vi "EnFlo_Tun_Heater_Control.vi"(1 "Ch Names":string[](array[string]), 2 "Heaters Just Enabled":bool, 3 "Values":dbl[](array[numeric]) format="%.2f") -> ()   [LabVIEW 2012]
uses:
  ADAM Client/Sub VIs/ADAM Controls/Search_mode.ctl
  ADAM_Global.vi
  <vilib>/Analysis/baseanly.llb/Mean (DBL).vi
  <vilib>/Analysis/NI_AALPro.lvlib
  <vilib>/Analysis/NI_AALBase.lvlib
panel:
  out "Read Values OK":bool
  out "History Out":dbl[](array[numeric])
  out "Current Temp":dbl
  out "Setpoint":dbl
  out "Large Error?":bool
  out "Error Range":dbl
  in  "Index To Display":i32
  in  "Derivative History Change":i32=60
  out "Feedback Temperature":string
  in  "Use Change Coeff if error above:":dbl=5.0 format="%_3g"
  in  "Minimum Power Change in %":dbl=0.08
  in  "Total History":i32=200
  out "Proportional Term":dbl format="%#.1f"
  out "Control Sum":dbl format="%#.1f"
  out "Differential Term":dbl format="%#.1f"
  in  "Derivative History":i32=60
  out "Integral Term":dbl format="%#.1f"
  # "This is the Max - Min error for the Total History"
  # "When Changing\nSetpoint"
  # "When running at\nSteady Cond"
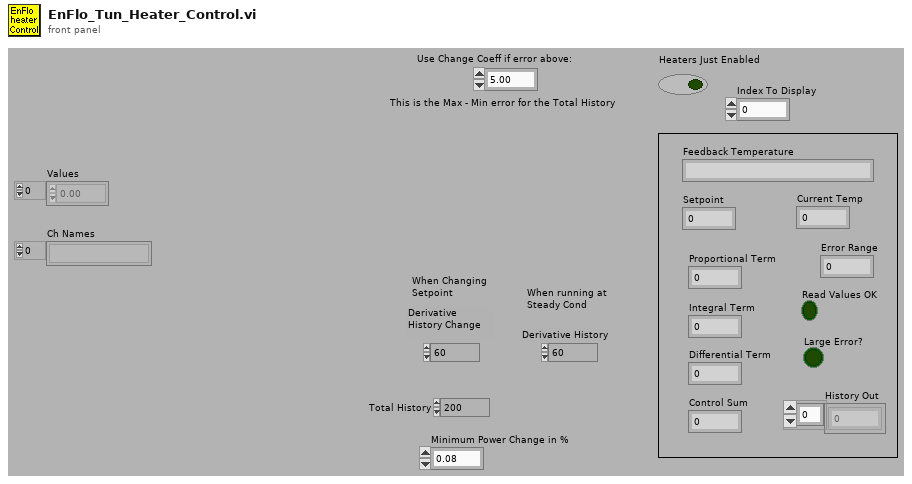
[diagram p1: front panel]
types:
  T1 = enum16{"On", "Off", "Always On", "Always Off", "Delete"}
  T2 = typedef "Search_mode.ctl" = enum16{"Between times", "All Times"}
  T3 = typedef "Ch_description_ADAM.ctl" = cluster{"Ch Name":string, "Type":T4, "Function":T5, "Ch State":T6, "Calibration type":T7, "A":dbl, "B":dbl, "C":dbl, "D":dbl, "Comments":string, "Address":T8, "String":string, "Duty":u16}
  T4 = typedef "Module_type_ADAM.ctl" = string
  T5 = typedef "Function_ADAM.ctl" = enum16{"Analogue Input", "Digital Input", "Event counter", "Event rate", "Analogue Output", "Digital Output", "Relay Output"}
  T6 = typedef "Channel_State.ctl" = enum16{"On", "Off", "Always On", "Always Off"}
  T7 = typedef "Calib_type_ADAM.ctl" = enum16{"Raw", "Bx + A", "Cx^2 + Bx + A", "Dx^3 + Cx^2 + Bx + A", "In Band", "Hi-Tec Q", "Hi-Tec M_dot", "Text"}
  T8 = typedef "Address.ctl" = cluster{"Main":i32, "Ch.":i32, "Sub":i32, "Port Name":string}
  T9 = cluster{"Centre Times":dbl[], "Output array":dbl[]}
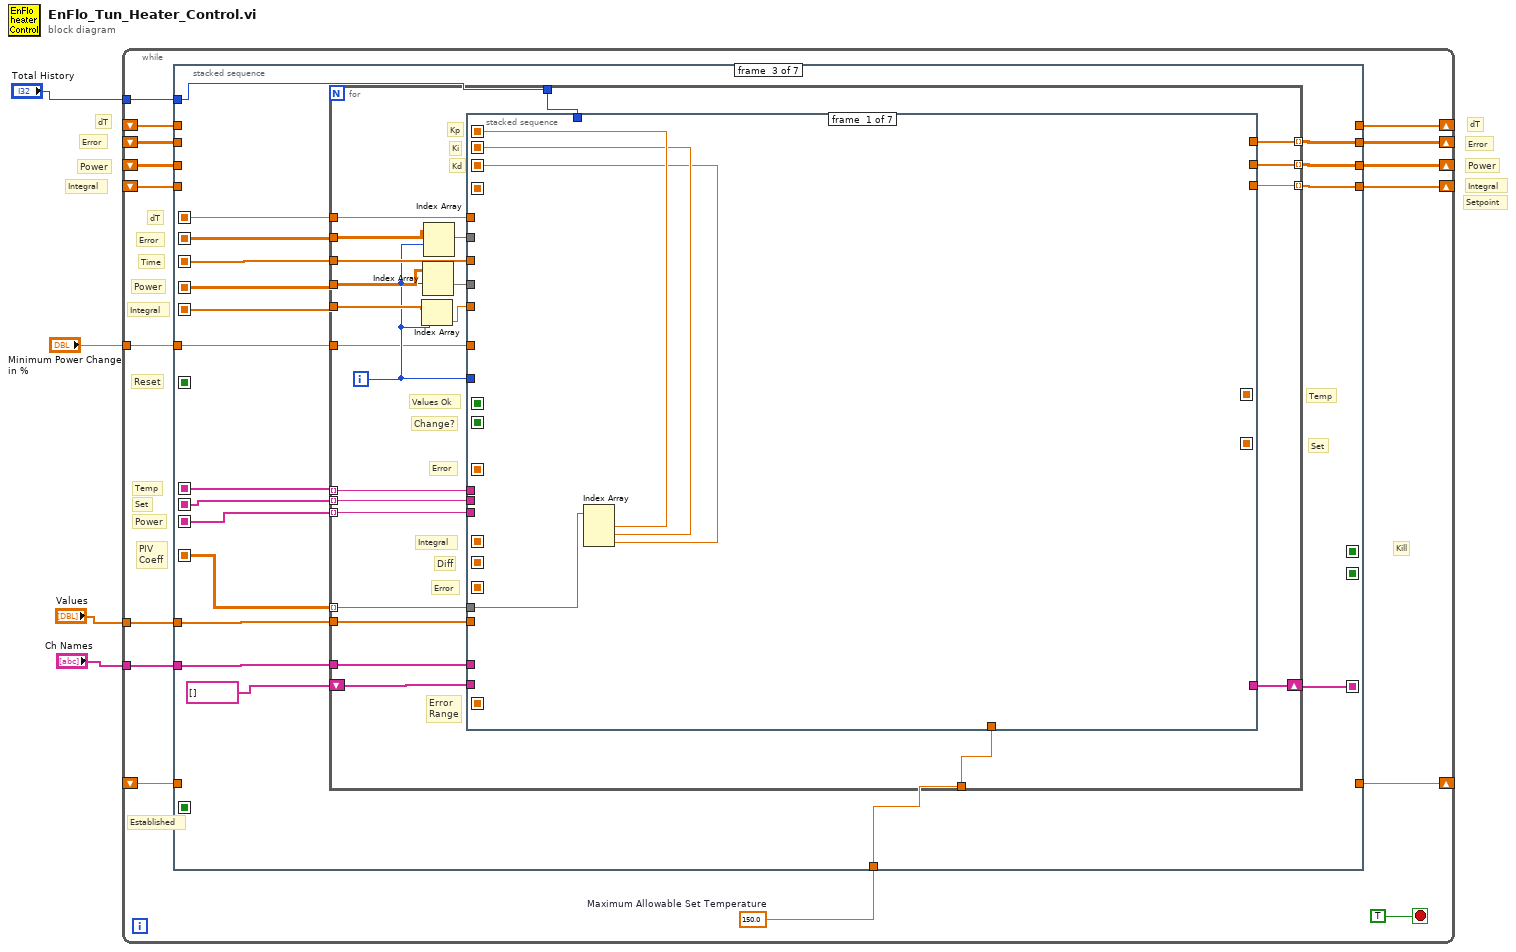
[diagram p0: block diagram]
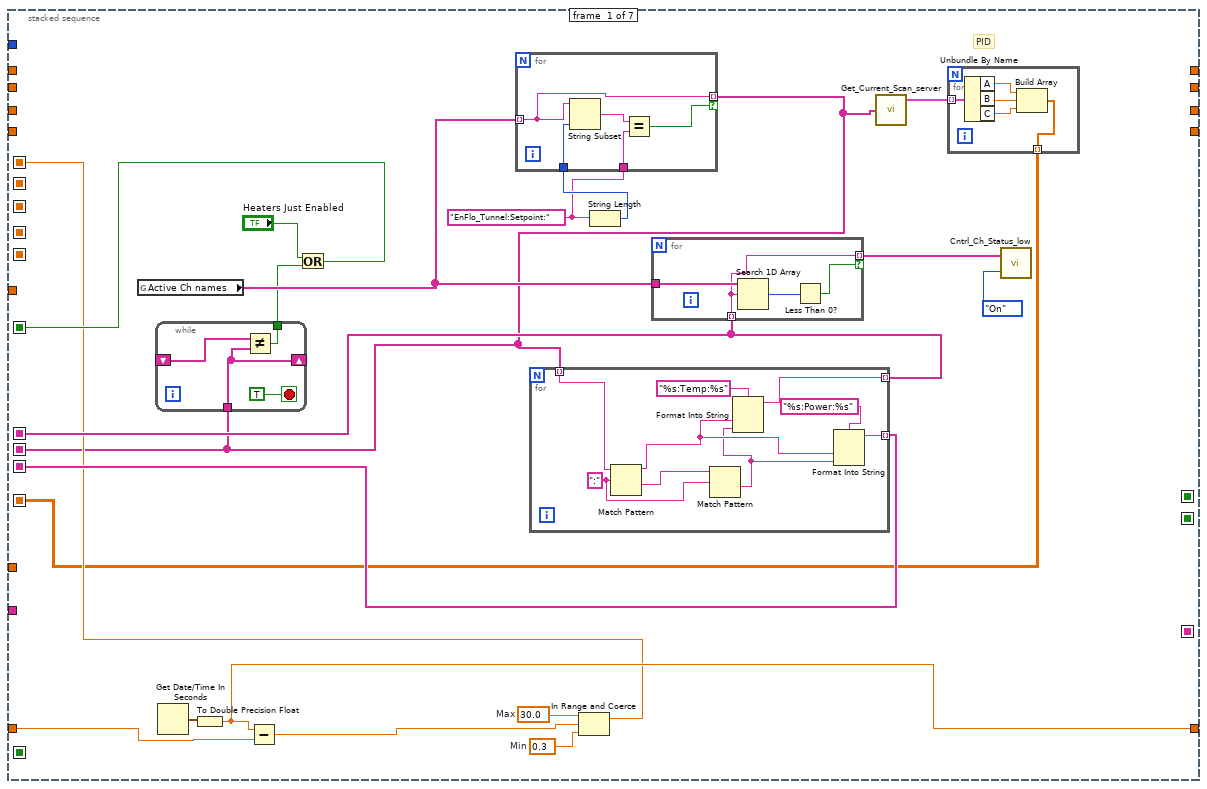
[diagram p2: hidden frame]
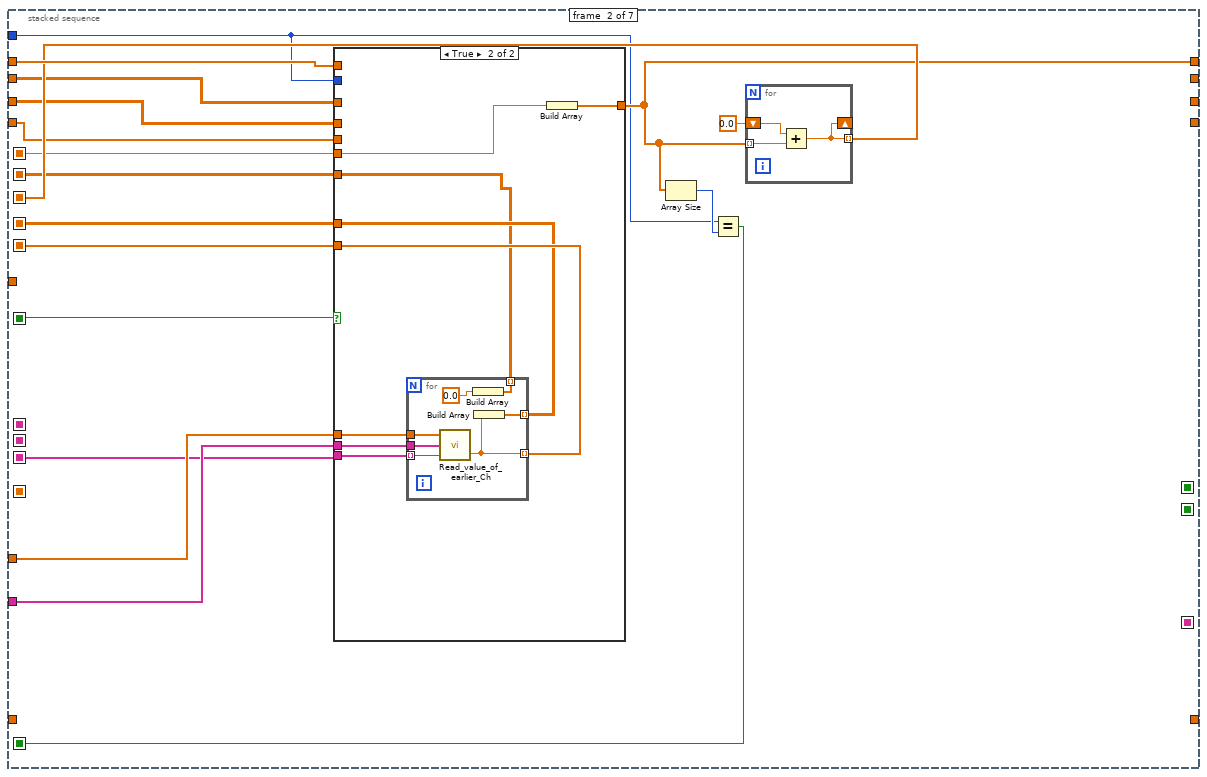
[diagram p3: hidden frame]
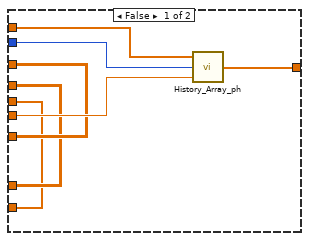
[diagram p4: hidden frame]
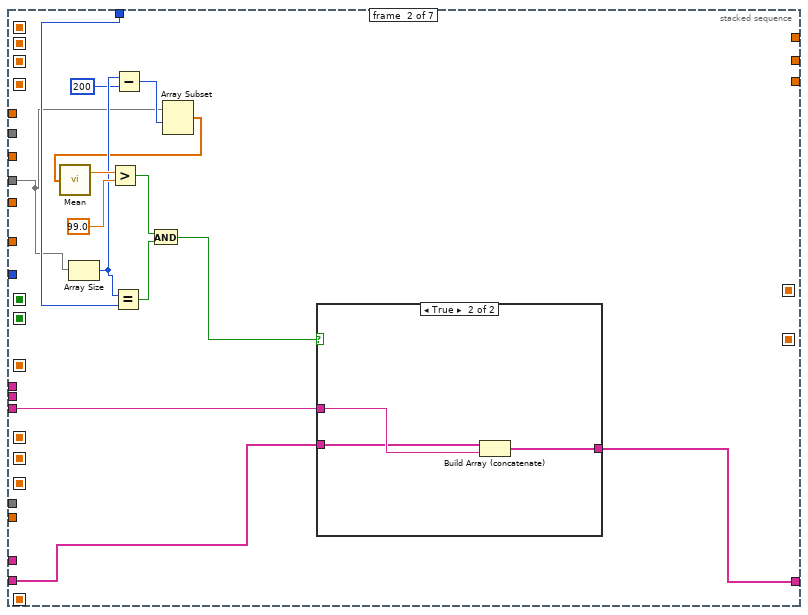
[diagram p5: hidden frame]
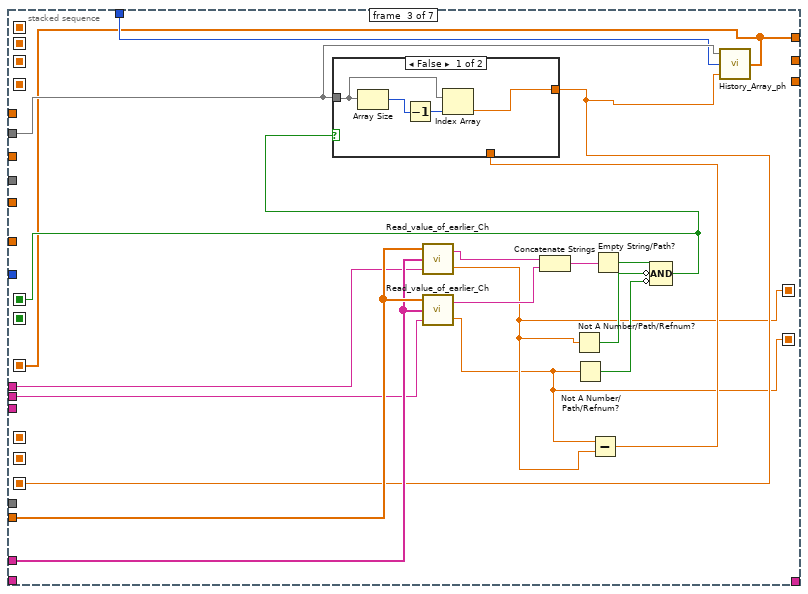
[diagram p7: hidden frame]
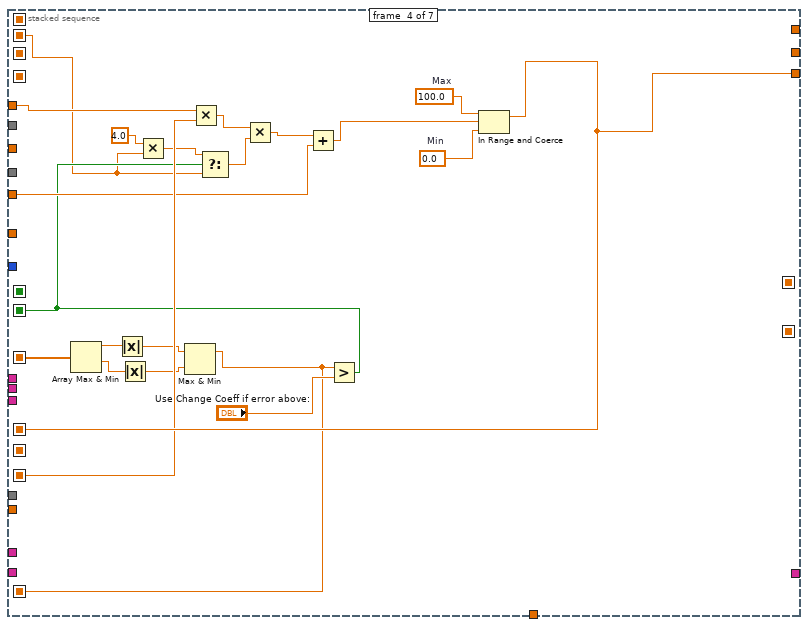
[diagram p9: hidden frame]
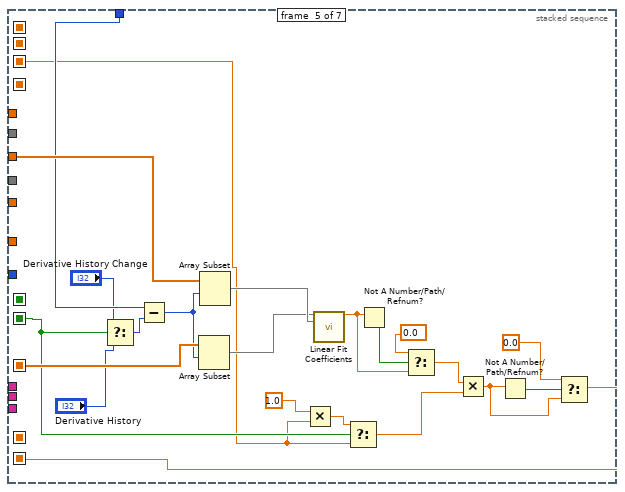
[diagram p10: hidden frame]
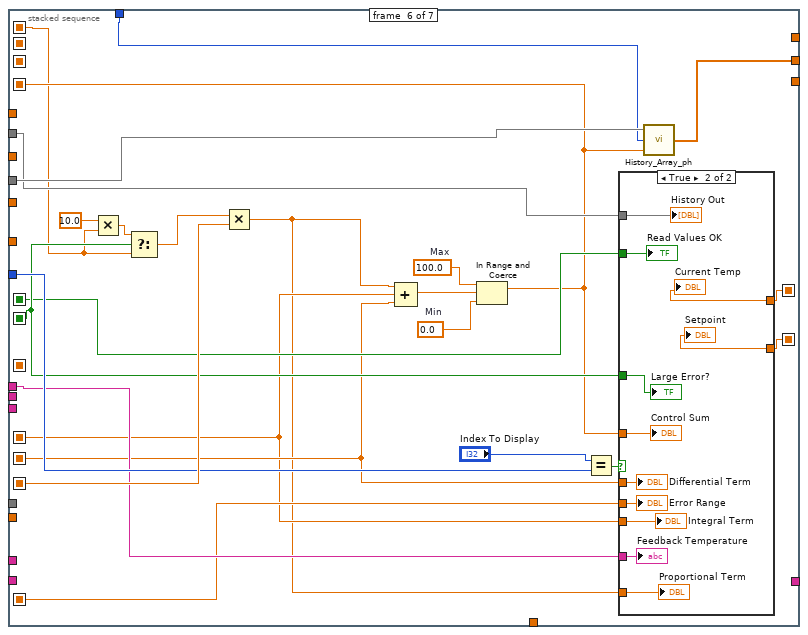
[diagram p11: hidden frame]
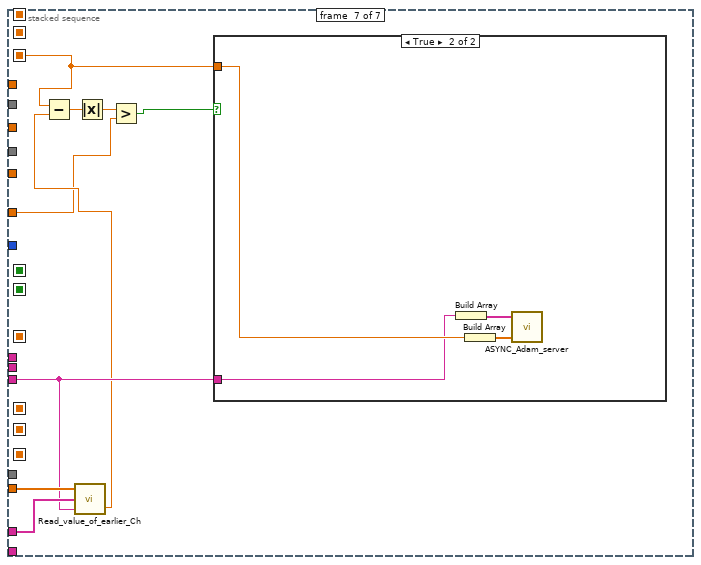
[diagram p13: hidden frame]
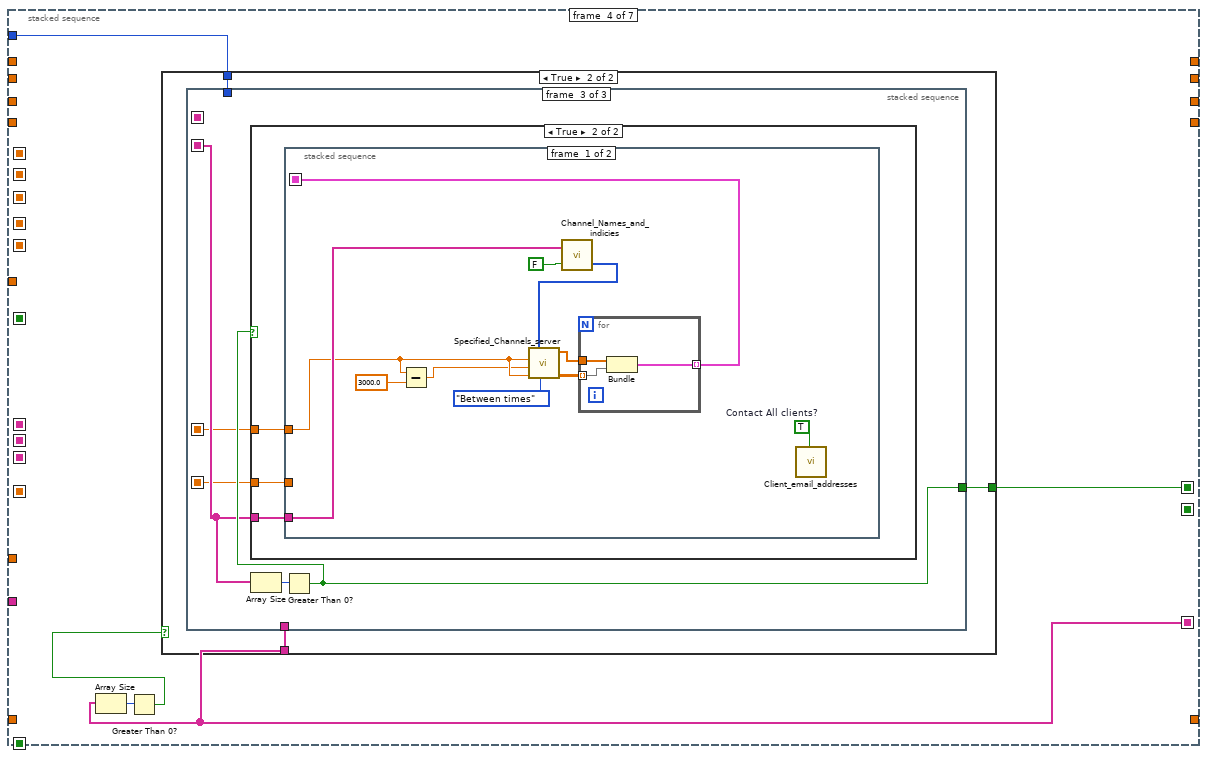
[diagram p15: hidden frame]
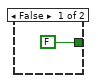
[diagram p16: hidden frame]
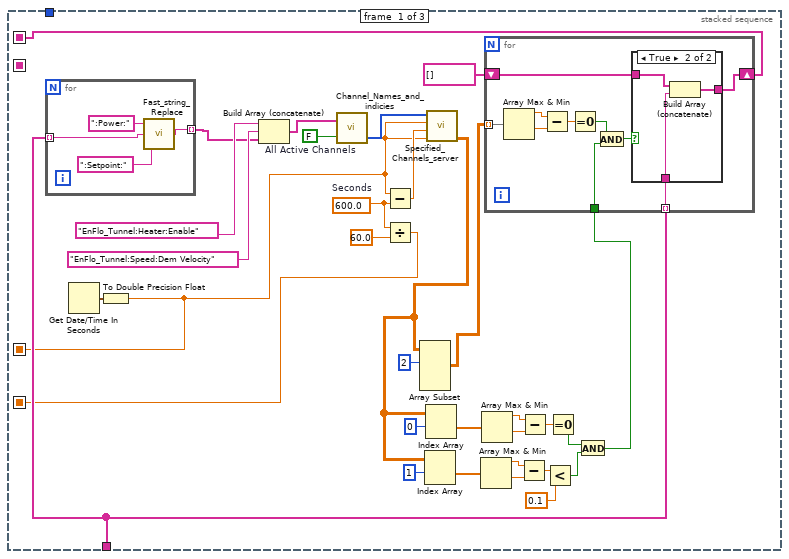
[diagram p17: hidden frame]
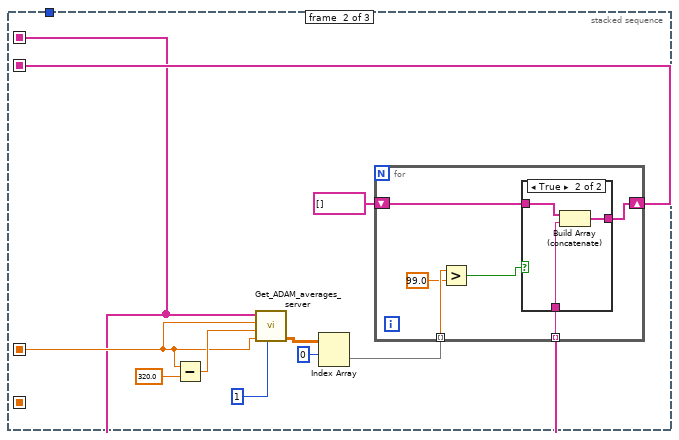
[diagram p19: hidden frame]
diagram:
  # "Integral"
  # "Power"
  # "Error"
  # "dT"
  # "Setpoint"
  # "Power"
  # "Integral"
  # "Error"
  # "dT"
  n1 = while {
    shift-right: [w18] -> _
    shift-left: _ -> [w19]
    shift-right: [w14] -> _
    shift-left: _ -> [w17]
    shift-right: [w16] -> _
    shift-left: _ -> [w15]
    shift-right: [w12] -> _
    shift-left: _ -> [w13]
    shift-right: [w10] -> _
    shift-left: _ -> [w11]
    tunnel: "Total History" -> [w9]
    tunnel: "Ch Names" -> [w7]
    tunnel: "Values" -> [w6]
    tunnel: "Minimum Power Change in %" -> [w5]
    stop <- TRUE stop-if-true
    w8 = 150.0  # Maximum Allowable Set Temperature
    # "Established"
    # "PIV\nCoeff"
    # "dT"
    # "Integral"
    # "Power"
    # "Error"
    # "Reset"
    # "Kill"
    # "Power"
    # "Set"
    # "Temp"
    # "Time"
    n2 = stacked-sequence {
      seq-local: [_ w82 _ _ _ _ _] -> [_ _ w128 _ _ _ _]
      seq-local: [w31 _ _ _ _ _ _] -> [_ _ w125 _ _ w452 _]
      seq-local: [w22 _ _ _ _ _ _] -> [_ _ w124 _ _ w451 _]
      seq-local: [w38 _ _ _ _ _ _] -> [_ w72 w123 _ _ w454 _]
      seq-local: [_ _ w120 _ _ _ _] -> [_ _ _ w292 _ _ _]
      seq-local: [_ _ _ w290 _ _ _] -> [_ _ _ _ w413 _ _]
      seq-local: [_ _ _ _ w414 _ _] -> [_ _ _ _ _ _ w495]
      seq-local: [w25 _ _ _ _ _ _] -> [_ w81 w116 _ _ _ _]
      seq-local: [w26 _ _ _ _ _ _] -> [_ w84 _ _ _ _ _]
      seq-local: [_ w80 _ _ _ _ _] -> [_ _ w113 _ _ _ _]
      seq-local: [_ w78 _ _ _ _ _] -> [_ _ w114 _ _ _ _]
      seq-local: [_ w76 _ _ _ _ _] -> [_ _ w115 _ _ _ _]
      seq-local: [w23 _ _ _ _ _ _] -> [_ _ w111 _ _ _ _]
      seq-local: [_ w68 _ _ _ _ _] -> [_ _ _ _ _ w443 _]
      tunnel: w19 -> [_ w85 _ _ _ _ _]
      tunnel: [_ w71 _ _ _ _ _] -> w18
      tunnel: w17 -> [_ w79 _ _ _ _ _]
      tunnel: [w32 _ _ _ _ _ _] -> w16
      tunnel: w15 -> [w34 _ _ _ _ _ _]
      tunnel: [_ _ w129 _ _ _ _] -> w14
      tunnel: w13 -> [_ w77 _ _ _ w453 _]
      tunnel: [_ _ w127 _ _ _ _] -> w12
      tunnel: w11 -> [_ w75 _ _ _ _ _]
      tunnel: [_ _ w126 _ _ _ _] -> w10
      tunnel: w9 -> [_ w69 w117 w293 w415 _ _]
      tunnel: w8 -> [_ _ w121 _ w407 _ _]
      tunnel: w7 -> [_ w73 w119 _ w410 w449 _]
      tunnel: w6 -> [_ w74 w118 _ w409 w450 _]
      tunnel: w5 -> [_ _ w112 _ _ w446 _]
      frame #0 {
        w36 = 0.3  # Min
        w35 = 30.0  # Max
        w39 = "EnFlo_Tunnel:Setpoint:"
        # "PID"
        n3 = global read "ADAM_Global.vi" "Active Ch names"() -> (w29:string[])
        n4 = Get Date/Time In Seconds() -> (seconds since 1Jan1904=w37:timestamp)
        n5 = To Double Precision Float(number=w37) -> (double precision float=w32:dbl)
        n6 = Subtract(x=w32, y=w34) -> (x-y=w33:dbl)
        n7 = In Range and Coerce(upper limit=w35, x=w33, lower limit=w36) -> (coerced(x)=w25:dbl)  [unwired: 1 out]
        n8 = String Length(string=w39) -> (length=w40:i32)
        n9 = for {
          tunnel: w29 -> [w55] mode=indexing
          tunnel: w40 -> [w58]
          tunnel: w39 -> [w57]
          tunnel: [w55] -> w22 mode=indexing if=w54
          n10 = String Subset(string=w55, length (rest)=w58) -> (substring=w56:string)  [unwired: 1 out]
          n11 = Equal?(x=w56, y=w57) -> (x = y?=w54:bool)
        }
        n12 = while {
          shift-right: [w49] -> _
          shift-left: _ -> [w48]
          tunnel: w22 -> [w49]
          tunnel: [w47] -> w27
          stop <- TRUE stop-if-true
          n13 = Not Equal?(x=w48, y=w49) -> (x != y?=w47:bool)
        }
        n14 = Or(x="Heaters Just Enabled", y=w27) -> (x .or. y?=w26:bool)
        n15 = for {
          tunnel: w22 -> [w59] mode=indexing
          tunnel: [w60] -> w38 mode=indexing
          tunnel: [w61] -> w31 mode=indexing
          w66 = ":" ("regular expression")
          n16 = Match Pattern(string=w59, regular expression=w66) -> (before substring=w63:string, after substring=w67:string)  [unwired: 3 out]
          n17 = Match Pattern(string=w67, regular expression=w66) -> (after substring=w62:string)  [unwired: 4 out]
          n18 = Format Into String(format string="%s:Temp:%s", w63, w62) -> (resulting string=w61:string)  [unwired: 2 in, 1 out]
          n19 = Format Into String(format string="%s:Power:%s", w63, w62) -> (resulting string=w60:string)  [unwired: 2 in, 1 out]
        }
        n20 = for {
          tunnel: w31 -> [w52] mode=indexing
          tunnel: w29 -> [w53]
          tunnel: [w52] -> w21 mode=indexing if=w50
          n21 = Search 1D Array(1D array=w53, element=w52) -> (index of element=w51:i32)  [unwired: 1 in]
          n22 = Less Than 0?(x=w51) -> (x < 0?=w50:bool)
        }
        n23 = call "Get_Current_Scan_server.vi"("Desired Channels"=w22) -> ("Ch Description Array"=w24:T3[])  [unwired: 2 out]
        n24 = for {
          tunnel: w24 -> [w45] mode=indexing
          tunnel: [w41] -> w23 mode=indexing
          n25 = Unbundle By Name(w45) -> ("A"=w44:dbl, "B"=w43:dbl, "C"=w42:dbl)
          n26 = Build Array(w44, w43, w42) -> (w41:dbl[])
        }
        n27 = call "Cntrl_Ch_Status_low.vi"("Mode"=T1."On", "Channel names"=w21) -> ()  [unwired: 1 out]
      }
      frame #1 {
        n28 = case shown="True" w84 {
          tunnel: [w95 w103] -> w71
          tunnel: w85 -> [w94 _]
          tunnel: w69 -> [w93 _]
          tunnel: w81 -> [w92 w102]
          tunnel: [w91 w96] -> w80
          tunnel: w79 -> [w91 _]
          tunnel: [w90 w97] -> w78
          tunnel: w77 -> [w90 _]
          tunnel: [w89 w98] -> w76
          tunnel: w75 -> [w89 _]
          tunnel: w74 -> [_ w101]
          tunnel: w73 -> [_ w100]
          tunnel: w72 -> [_ w99]
          frame False {
            n29 = call "History_Array_ph.vi"("Current Value"=w92, "Desired Length"=w93, "History In"=w94) -> ("History Out"=w95:dbl[])
          }
          frame True {
            n30 = for {
              tunnel: w101 -> [w110]
              tunnel: w100 -> [w109]
              tunnel: w99 -> [w108] mode=indexing
              tunnel: [w104] -> w98 mode=indexing
              tunnel: [w107] -> w97 mode=indexing
              tunnel: [w105] -> w96 mode=indexing
              n31 = call "Read_value_of_earlier_Ch.vi"("Desired Ch to Read"=w108, "Ch names"=w109, "Present scan array"=w110) -> ("Value"=w104:dbl)  [unwired: 1 in, 1 out]
              n32 = Build Array(0.0) -> (w105:dbl[])
              n33 = Build Array(w104) -> (w107:dbl[])
            }
            n34 = Build Array(w102) -> (w103:dbl[])
          }
        }
        n35 = Array Size(array=w71) -> (size(s)=w70:i32)
        n36 = Equal?(x=w69, y=w70) -> (x = y?=w68:bool)
        n37 = for {
          shift-right: [w87] -> _
          shift-left: 0.0 ("element") -> [w88]
          tunnel: [w87] -> w82 mode=indexing
          tunnel: w71 -> [w86] mode=indexing
          n38 = Add(x=w88, y=w86) -> (x+y=w87:dbl)
        }
      }
      frame #2 {
        # "Temp"
        # "Set"
        n39 = for {
          tunnel: w118 -> [w137]
          tunnel: w119 -> [w136]
          tunnel: [w152] -> w129 mode=indexing
          tunnel: w113 -> [w140]
          tunnel: w116 -> [w151]
          tunnel: w128 -> [w142]
          tunnel: [w150] -> w127 mode=indexing
          tunnel: w114 -> [w141]
          tunnel: [w149] -> w126 mode=indexing
          tunnel: w115 -> [w143]
          tunnel: w125 -> [w148] mode=indexing
          tunnel: w124 -> [w135] mode=indexing
          tunnel: w123 -> [w147] mode=indexing
          shift-right: [w145] -> w120
          shift-left: string[] [] -> [w146]
          tunnel: w121 -> [w144]
          tunnel: w117 -> [w139]
          tunnel: w112 -> [w131]
          tunnel: w111 -> [w130] mode=indexing
          i -> [w138]
          # "Kd"
          # "Ki"
          # "Kp"
          # "Values Ok"
          # "Error\nRange"
          # "Change?"
          # "Integral"
          # "Error"
          # "Error"
          # "Diff"
          n40 = Index Array(array=w143, index=w138) -> (element=w134:dbl)
          n41 = Index Array(array=w141, index (row)=w138) -> (element=w132:dbl[])  [unwired: 1 in]
          n42 = Index Array(array=w140, index (row)=w138) -> (element=w133:dbl[])  [unwired: 1 in]
          n43 = stacked-sequence {
            seq-local: [_ _ _ _ w235 _ _] -> [_ _ _ _ _ w246 _]
            seq-local: [_ _ w178 _ _ _ _] -> [_ _ _ w217 _ w265 _]
            seq-local: [_ _ w177 _ _ _ _] -> [_ _ _ w215 w230 _ _]
            seq-local: [_ _ _ w218 _ _ _] -> [_ _ _ _ _ w245 _]
            seq-local: [_ _ _ _ _ w247 _] -> [_ _ _ _ _ _ w282]
            seq-local: [_ _ w179 _ _ _ _] -> [_ _ _ _ _ w248 _]
            seq-local: [_ _ _ w213 _ _ _] -> [_ _ _ _ w225 w252 _]
            seq-local: [_ _ _ w202 _ _ _] -> [_ _ _ _ _ w253 _]
            seq-local: [_ _ w176 _ _ _ _] -> [_ _ _ _ _ w250 _]
            seq-local: [_ _ w175 _ _ _ _] -> [_ _ _ _ _ w251 _]
            seq-local: [w155 _ _ _ _ _ _] -> [_ _ _ _ _ w243 _]
            seq-local: [w154 _ _ _ _ _ _] -> [_ _ _ w200 _ _ _]
            seq-local: [w153 _ _ _ _ _ _] -> [_ _ _ _ w221 _ _]
            tunnel: w137 -> [_ _ w192 _ _ _ w285]
            tunnel: w136 -> [_ _ w191 _ _ _ w284]
            tunnel: [_ _ w177 _ _ _ _] -> w152
            tunnel: w133 -> [_ _ w181 _ _ w249 _]
            tunnel: w151 -> [_ _ _ w201 _ _ _]
            tunnel: w142 -> [_ _ _ _ w232 _ _]
            tunnel: [_ _ _ _ _ w261 _] -> w150
            tunnel: w132 -> [_ w158 _ _ _ w260 _]
            tunnel: [_ _ _ w218 _ _ _] -> w149
            tunnel: w134 -> [_ _ _ w216 _ _ _]
            tunnel: w148 -> [_ _ w182 _ _ w254 _]
            tunnel: w135 -> [_ _ w183 _ _ _ _]
            tunnel: w147 -> [_ w165 _ _ _ _ w283]
            tunnel: w146 -> [_ w164 _ _ _ _ _]
            tunnel: [_ w163 _ _ _ _ _] -> w145
            tunnel: w144 -> [_ _ _ _ _ _ _]
            tunnel: w139 -> [_ w162 w180 _ w227 w259 _]
            tunnel: w138 -> [_ _ _ _ _ w256 _]
            tunnel: w131 -> [_ _ _ _ _ _ w277]
            tunnel: w130 -> [w156 _ _ _ _ _ _]
            frame #0 {
              n44 = Index Array(array=w156) -> (element #1=w155:dbl, element #2=w154:dbl, element #3=w153:dbl)  [unwired: 3 in]
            }
            frame #1 {
              n45 = Array Size(array=w158) -> (size(s)=w161:i32)
              n46 = Equal?(x=w161, y=w162) -> (x = y?=w168:bool)
              n47 = Subtract(x=w161, y=200) -> (x-y=w159:i32)
              n48 = Array Subset(array=w158, index=w159) -> (w157:dbl[])  [unwired: 1 in]
              n49 = call-poly <vilib>:"Mean.vi"("X"=w157) -> ("mean"=w170:dbl)  [unwired: 1 out]
              n50 = Greater?(x=w170, y=99.0) -> (0:w167:bool)
              n51 = And(x=w167, y=w168) -> (x .and. y?=w166:bool)
              n52 = case shown="True" w166 {
                tunnel: w165 -> [_ w174]
                tunnel: w164 -> [w171 w173]
                tunnel: [w171 w172] -> w163
                frame False {
                }
                frame True {
                  n53 = Build Array (concatenate)(w173, w174) -> (w172:string[])
                }
              }
            }
            frame #2 {
              n54 = call "Read_value_of_earlier_Ch.vi"("Desired Ch to Read"=w182, "Ch names"=w191, "Present scan array"=w192) -> ("Value"=w176:dbl, "Scan comment"=w190:string)  [unwired: 1 in]
              n55 = call "Read_value_of_earlier_Ch.vi"("Desired Ch to Read"=w183, "Ch names"=w191, "Present scan array"=w192) -> ("Value"=w175:dbl, "Scan comment"=w189:string)  [unwired: 1 in]
              n56 = Concatenate Strings(w190, w189) -> (w188:string)
              n57 = Not A Number/Path/Refnum?(number/path/refnum=w176) -> (NaN/Path/Refnum?=w186:bool)
              n58 = Not A Number/Path/Refnum?(number/path/refnum=w175) -> (NaN/Path/Refnum?=w185:bool)
              n59 = Subtract(x=w175, y=w176) -> (x-y=w184:dbl)
              n60 = Empty String/Path?(string/path=w188) -> (empty?=w187:bool)
              n61 = Compound Arithmetic op=AND(w187, invert w186, invert w185) -> (w179:bool)
              n62 = case shown="False" w179 {
                tunnel: w181 -> [w193 _]
                tunnel: [w196 w197] -> w178
                tunnel: w184 -> [_ w197]
                frame False {
                  n63 = Array Size(array=w193) -> (size(s)=w194:i32)
                  n64 = Decrement(x=w194) -> (x-1=w195:i32)
                  n65 = Index Array(array=w193, index=w195) -> (element=w196:dbl)
                }
                frame True {
                }
              }
              n66 = call "History_Array_ph.vi"("Current Value"=w178, "Desired Length"=w180, "History In"=w181) -> ("History Out"=w177:dbl[])
            }
            frame #3 {
              w212 = 0.0  # Min
              w211 = 100.0  # Max
              n67 = Array Max & Min(array=w215) -> (max value=w206:dbl, min value=w205:dbl)  [unwired: 2 out]
              n68 = Absolute Value(x=w206) -> (abs(x)=w203:dbl)
              n69 = Absolute Value(x=w205) -> (abs(x)=w204:dbl)
              n70 = Multiply(x=4.0, y=w200) -> (x*y=w198:dbl)
              n71 = Max & Min(x=w203, y=w204) -> (max(x,y)=w202:dbl)  [unwired: 1 out]
              n72 = Multiply(x=w201, y=w217) -> (x*y=w210:dbl)
              n73 = Greater?(x=w202, y="Use Change Coeff if error above:") -> (0:w213:bool)
              n74 = Select(t=w198, s=w213, f=w200) -> (s? t:f=w207:dbl)
              n75 = Multiply(x=w210, y=w207) -> (x*y=w209:dbl)
              n76 = Add(x=w209, y=w216) -> (x+y=w208:dbl)
              n77 = In Range and Coerce(upper limit=w211, x=w208, lower limit=w212) -> (coerced(x)=w218:dbl)  [unwired: 1 out]
            }
            frame #4 {
              n78 = Select(t="Derivative History Change", s=w225, f="Derivative History") -> (s? t:f=w222:i32)
              n79 = Subtract(x=w227, y=w222) -> (x-y=w228:i32)
              n80 = Array Subset(array=w230, index=w228) -> (w229:dbl[])  [unwired: 1 in]
              n81 = Array Subset(array=w232, index=w228) -> (w231:dbl[])  [unwired: 1 in]
              n82 = Multiply(x=1.0, y=w221) -> (x*y=w220:dbl)
              n83 = call <vilib>:"Linear Fit Coefficients.vi"("Y"=w229, "X"=w231) -> ("slope"=w240:dbl)  [unwired: 3 in, 10 out]
              n84 = Select(t=w220, s=w225, f=w221) -> (s? t:f=w226:dbl)
              n85 = Not A Number/Path/Refnum?(number/path/refnum=w240) -> (NaN/Path/Refnum?=w238:bool)
              n86 = Select(t=0.0 ("f"), s=w238, f=w240) -> (s? t:f=w237:dbl)
              n87 = Multiply(x=w237, y=w226) -> (x*y=w234:dbl)
              n88 = Not A Number/Path/Refnum?(number/path/refnum=w234) -> (NaN/Path/Refnum?=w236:bool)
              n89 = Select(t=0.0, s=w236, f=w234) -> (s? t:f=w235:dbl)
            }
            frame #5 {
              w264 = 0.0  # Min
              w263 = 100.0  # Max
              n90 = Multiply(x=10.0, y=w243) -> (x*y=w242:dbl)
              n91 = Select(t=w242, s=w252, f=w243) -> (s? t:f=w258:dbl)
              n92 = Multiply(x=w258, y=w265) -> (x*y=w244:dbl)
              n93 = Compound Arithmetic op=ADD(w244, w245, w246) -> (w262:dbl)
              n94 = In Range and Coerce(upper limit=w263, x=w262, lower limit=w264) -> (coerced(x)=w247:dbl)  [unwired: 1 out]
              n95 = Equal?(x="Index To Display", y=w256) -> (x = y?=w255:bool)
              n96 = case shown="True" w255 {
                tunnel: w244 -> [_ w276]
                tunnel: w247 -> [_ w275]
                tunnel: w246 -> [_ w274]
                tunnel: w245 -> [_ w273]
                tunnel: w254 -> [_ w272]
                tunnel: w253 -> [_ w271]
                tunnel: w252 -> [_ w270]
                tunnel: w251 -> [_ w269]
                tunnel: w250 -> [_ w268]
                tunnel: w249 -> [_ w267]
                tunnel: w248 -> [_ w266]
                frame False {
                }
                frame True {
                  "Control Sum" <- w275
                  "Proportional Term" <- w276
                  "Differential Term" <- w274
                  "Integral Term" <- w273
                  "Feedback Temperature" <- w272
                  "Error Range" <- w271
                  "Large Error?" <- w270
                  "Setpoint" <- w269
                  "Current Temp" <- w268
                  "History Out" <- w267
                  "Read Values OK" <- w266
                }
              }
              n97 = call "History_Array_ph.vi"("Current Value"=w247, "Desired Length"=w259, "History In"=w260) -> ("History Out"=w261:dbl[])
            }
            frame #6 {
              n98 = call "Read_value_of_earlier_Ch.vi"("Desired Ch to Read"=w283, "Ch names"=w284, "Present scan array"=w285) -> ("Value"=w281:dbl)  [unwired: 1 in, 1 out]
              n99 = Subtract(x=w282, y=w281) -> (x-y=w280:dbl)
              n100 = Absolute Value(x=w280) -> (abs(x)=w279:dbl)
              n101 = Greater?(x=w279, y=w277) -> (0:w278:bool)
              n102 = case shown="True" w278 {
                tunnel: w282 -> [_ w287]
                tunnel: w283 -> [_ w286]
                frame False {
                }
                frame True {
                  n103 = Build Array(w286) -> (w288:string[])
                  n104 = Build Array(w287) -> (w289:dbl[])
                  n105 = call "ASYNC_Adam_server.vi"("Values"=w289, "Channel Names"=w288) -> ()  [unwired: 1 in, 3 out]
                }
              }
            }
          }
        }
      }
      frame #3 {
        n106 = Array Size(array=w292) -> (size(s)=w294:i32)
        n107 = Greater Than 0?(x=w294) -> (x > 0?=w291:bool)
        n108 = case shown="True" w291 {
          tunnel: w293 -> [_ w297]
          tunnel: w292 -> [_ w298]
          tunnel: [FALSE w296] -> w290
          frame False {
          }
          frame True {
            n109 = stacked-sequence {
              seq-local: [w326 _ _] -> [_ w350 _]
              seq-local: [w302 _ _] -> [_ w356 w370]
              seq-local: [_ w351 _] -> [_ _ w371]
              seq-local: [w299 _ _] -> [_ _ w369]
              tunnel: w298 -> [w325 _ _]
              tunnel: w297 -> [_ _ _]
              tunnel: [_ _ w372] -> w296
              frame #0 {
                w301 = 600.0  # Seconds
                w330 = FALSE  # All Active Channels
                n110 = for {
                  tunnel: w325 -> [w346] mode=indexing
                  tunnel: [w345] -> w303 mode=indexing
                  n111 = call "Fast_string_Replace.vi"("Replace match with:"=":Setpoint:" ("regular expression"), "Input String"=w346, "regular expression"=":Power:") -> ("Output String"=w345:string)  [unwired: 2 out]
                }
                n112 = Get Date/Time In Seconds() -> (seconds since 1Jan1904=w328:timestamp)
                n113 = To Double Precision Float(number=w328) -> (double precision float=w302:dbl)
                n114 = Build Array (concatenate)("EnFlo_Tunnel:Heater:Enable", "EnFlo_Tunnel:Speed:Dem Velocity", w303) -> (w322:string[])
                n115 = call "Channel_Names_and_indicies.vi"("All Active Channels"=w330, "Desired Ch Names"=w322) -> ("Indicies"=w329:i32[])  [unwired: 1 out]
                n116 = Subtract(x=w302, y=w301) -> (x-y=w324:dbl)
                n117 = Divide(x=w301, y=60.0) -> (x/y=w299:dbl)
                n118 = call "Specified_Channels_server.vi"("End time"=w302, "Start time"=w324, "Clients time"=w302, "Requested channels"=w329) -> ("Output array"=w309:dbl[][])  [unwired: 1 in, 4 out]
                n119 = Array Subset(array=w309, index (row)=2 ("index")) -> (w320:dbl[][])  [unwired: 3 in]
                n120 = Index Array(array=w309, index (row)=1) -> (element=w314:dbl[])  [unwired: 1 in]
                n121 = Index Array(array=w309, index (row)=0) -> (element=w316:dbl[])  [unwired: 1 in]
                n122 = Array Max & Min(array=w314) -> (max value=w312:dbl, min value=w313:dbl)  [unwired: 2 out]
                n123 = Array Max & Min(array=w316) -> (max value=w318:dbl, min value=w317:dbl)  [unwired: 2 out]
                n124 = Subtract(x=w312, y=w313) -> (x-y=w306:dbl)
                n125 = Subtract(x=w318, y=w317) -> (x-y=w319:dbl)
                n126 = Less?(x=w306, y=0.1) -> (x < y?=w304:bool)
                n127 = Equal To 0?(x=w319) -> (x = 0?=w308:bool)
                n128 = And(x=w308, y=w304) -> (x .and. y?=w307:bool)
                n129 = for {
                  tunnel: w320 -> [w340] mode=indexing
                  shift-right: [w334] -> w326
                  shift-left: string[] [] -> [w335]
                  tunnel: w325 -> [w336] mode=indexing
                  tunnel: w307 -> [w331]
                  n130 = Array Max & Min(array=w340) -> (max value=w338:dbl, min value=w339:dbl)  [unwired: 2 out]
                  n131 = Subtract(x=w338, y=w339) -> (x-y=w337:dbl)
                  n132 = Equal To 0?(x=w337) -> (x = 0?=w333:bool)
                  n133 = And(x=w333, y=w331) -> (x .and. y?=w332:bool)
                  n134 = case shown="True" w332 {
                    tunnel: w336 -> [_ w344]
                    tunnel: w335 -> [w341 w343]
                    tunnel: [w341 w342] -> w334
                    frame False {
                    }
                    frame True {
                      n135 = Build Array (concatenate)(w343, w344) -> (w342:string[])
                    }
                  }
                }
              }
              frame #1 {
                n136 = Subtract(x=w356, y=320.0) -> (x-y=w357:dbl)
                n137 = call "Get_ADAM_averages_server.vi"("No of averages"=1, "End time"=w356, "Start time"=w357, "Clients time"=w356, "ADAM Ch Names"=w350) -> ("DBL values"=w354:dbl[][])  [unwired: 1 in, 4 out]
                n138 = Index Array(array=w354, index (row)=0) -> (element=w352:dbl[])  [unwired: 1 in]
                n139 = for {
                  shift-right: [w363] -> w351
                  shift-left: string[] [] -> [w359]
                  tunnel: w350 -> [w364] mode=indexing
                  tunnel: w352 -> [w362] mode=indexing
                  n140 = Greater?(x=w362, y=99.0) -> (0:w360:bool)
                  n141 = case shown="True" w360 {
                    tunnel: w364 -> [_ w368]
                    tunnel: w359 -> [w365 w367]
                    tunnel: [w365 w366] -> w363
                    frame False {
                    }
                    frame True {
                      n142 = Build Array (concatenate)(w367, w368) -> (w366:string[])
                    }
                  }
                }
              }
              frame #2 {
                n143 = Array Size(array=w371) -> (size(s)=w373:i32)
                n144 = Greater Than 0?(x=w373) -> (x > 0?=w372:bool)
                n145 = case shown="True" w372 {
                  tunnel: w371 -> [_ w376]
                  tunnel: w370 -> [_ w375]
                  tunnel: w369 -> [_ w374]
                  frame False {
                  }
                  frame True {
                    n146 = stacked-sequence {
                      seq-local: [w378 _] -> [_ w394]
                      tunnel: w376 -> [w383 w396]
                      tunnel: w375 -> [w382 _]
                      tunnel: w374 -> [_ w391]
                      frame #0 {
                        w377 = TRUE  # Contact All clients?
                        n147 = Subtract(x=w382, y=3000.0) -> (x-y=w380:dbl)
                        n148 = call "Channel_Names_and_indicies.vi"("All Active Channels"=FALSE, "Desired Ch Names"=w383) -> ("Indicies"=w386:i32[])  [unwired: 1 out]
                        n149 = call "Specified_Channels_server.vi"("Mode"=Search_mode."Between times", "End time"=w382, "Start time"=w380, "Clients time"=w382, "Requested channels"=w386) -> ("Output array"=w379:dbl[][], "Centre Times"=w387:dbl[])  [unwired: 3 out]
                        n150 = for {
                          tunnel: w387 -> [w390]
                          tunnel: w379 -> [w389] mode=indexing
                          tunnel: [w388] -> w378 mode=indexing
                          n151 = Bundle("Centre Times"=w390, "Output array"=w389) -> (w388:T9)  [unwired: 1 out]
                        }
                        n152 = call "Client_email_addresses.vi"("Contact All clients?"=w377) -> ()  [unwired: 2 in]
                      }
                      frame #1 {
                        n153 = for {
                          shift-right: [w401] -> w392
                          shift-left: "" -> [w404]
                          tunnel: w396 -> [w402] mode=indexing
                          n154 = Concatenate Strings(w404, w402, "\r\n") -> (w401:string)
                        }
                        n155 = Format Into String(format string="The following channels have been at 100%% Power for %d minutes\n\n%s\n\n\"EnFlo_Tunnel:Heater:Enable\" has therefore been set to 0", w391, w392) -> (resulting string=w397:string)  [unwired: 2 in, 1 out]
                        n156 = call "Email_Attachment_Plot.vi"("X axis name"="Time", "Y axis name"="Power (%)", "XY Graph"=w394, "Series Names"=w396, "message"=w397, "subject ([No Subject])"="Heater Shutdown" ("t")) -> ()  [unwired: 1 out]
                      }
                    }
                  }
                }
              }
            }
          }
        }
      }
      frame #4 {
        w411 = "EnFlo_Tunnel:Temp:"
        n157 = String Length(string=w411) -> (length=w412:i32)
        n158 = for {
          shift-right: [w421] -> w405
          shift-left: "" -> [w422]
          tunnel: w410 -> [w425] mode=indexing
          tunnel: w412 -> [w426]
          tunnel: w411 -> [w423]
          tunnel: w409 -> [w420] mode=indexing
          tunnel: w407 -> [w419]
          n159 = String Subset(string=w425, length (rest)=w426) -> (substring=w424:string)  [unwired: 1 out]
          n160 = Equal?(x=w424, y=w423) -> (x = y?=w416:bool)
          n161 = Greater?(x=w420, y=w419) -> (0:w417:bool)
          n162 = And(x=w416, y=w417) -> (x .and. y?=w418:bool)
          n163 = case shown="True" w418 {
            tunnel: w425 -> [_ w428]
            tunnel: w422 -> [w427 w430]
            tunnel: [w427 w429] -> w421
            frame False {
            }
            frame True {
              n164 = Concatenate Strings(w430, w428, "\r\n") -> (w429:string)
            }
          }
        }
        n165 = Empty String/Path?(string/path=w405) -> (empty?=w406:bool)
        n166 = case shown="False" w406 {
          tunnel: w415 -> [_ _]
          tunnel: w407 -> [w433 _]
          tunnel: [TRUE w439] -> w414
          tunnel: w413 -> [_ w439]
          tunnel: w405 -> [w432 _]
          frame False {
            n167 = Format Into String(format string="The following channels have reached a temperature of  %d deg C\n\n%s\n\n\"EnFlo_Tunnel:Heater:Enable\" has therefore been set to 0", w433, w432) -> (resulting string=w435:string)  [unwired: 2 in, 1 out]
            n168 = call "Server_Emails.vi"("Client Name Contains"="EnFlo_Tunnel", "Message"=w435, "Subject"="Heater Shutdown" ("t")) -> ()  [unwired: 2 in, 3 out]
          }
          frame True {
          }
        }
      }
      frame #5 {
        w447 = ""
        # "Integer Precision on measure temp\nso that not too many emails are sent"
        n169 = Add(x=w446, y=0.2) -> (x+y=w444:dbl)
        n170 = for {
          tunnel: w454 -> [w474] mode=indexing
          tunnel: w453 -> [w479] mode=indexing
          shift-right: [w475] -> w448
          shift-left: w447 -> [w476]
          tunnel: w452 -> [w473] mode=indexing
          tunnel: w451 -> [w472] mode=indexing
          tunnel: w450 -> [w471]
          tunnel: w449 -> [w470]
          shift-right: [w468] -> w442
          shift-left: w447 -> [w469]
          tunnel: w444 -> [w467]
          n171 = call-poly <vilib>:"Mean.vi"("X"=w479) -> ("mean"=w478:dbl)  [unwired: 1 out]
          n172 = Greater?(x=w478, y=w467) -> (0:w477:bool)
          n173 = case shown="False" w477 {
            tunnel: w476 -> [w488 w494]
            tunnel: [w487 w494] -> w475
            tunnel: w474 -> [w485 _]
            tunnel: w473 -> [w492 _]
            tunnel: w472 -> [w491 _]
            tunnel: w471 -> [w490 _]
            tunnel: w470 -> [w489 _]
            tunnel: w469 -> [w482 w493]
            tunnel: [w481 w493] -> w468
            frame False {
              n174 = call "Read_value_of_earlier_Ch.vi"("Desired Ch to Read"=w492, "Ch names"=w489, "Present scan array"=w490) -> ("Value"=w483:dbl)  [unwired: 1 in, 1 out]
              n175 = call "Read_value_of_earlier_Ch.vi"("Desired Ch to Read"=w491, "Ch names"=w489, "Present scan array"=w490) -> ("Value"=w484:dbl)  [unwired: 1 in, 1 out]
              n176 = Format Into String(format string="%s has a setpoint temp of %.1f and a measured temp of %.1f.\n", initial string=w488, w485, w484, w483) -> (resulting string=w487:string)  [unwired: 1 in, 1 out]
              n177 = Format Into String(format string="%s has a setpoint temp of %.1f and a measured temp of %d.\n", initial string=w482, w485, w484, w483) -> (resulting string=w481:string)  [unwired: 1 in, 1 out]
            }
            frame True {
            }
          }
        }
        n178 = Select(t=w442, s=w443, f="") -> (s? t:f=w440:string)
        n179 = while {
          tunnel: w448 -> [w458]
          shift-right: [w455] -> _
          shift-left: _ -> [w456]
          tunnel: w440 -> [w455]
          stop <- TRUE stop-if-true
          n180 = Not Equal?(x=w455, y=w456) -> (x != y?=w460:bool)
          n181 = Empty String/Path?(string/path=w455) -> (empty?=w459:bool)
          n182 = Compound Arithmetic op=AND(w460, invert w459) -> (w457:bool)
          n183 = case shown="True" w457 {
            tunnel: w458 -> [_ w463]
            frame False {
            }
            frame True {
              n184 = Format Into String(format string="The following channels have currently have a zero power demand:\n\n%s\n\n \nPlease check that this is not adversly affecting your experimental conditions.", w463) -> (resulting string=w462:string)  [unwired: 2 in, 1 out]
              n185 = call "Server_Emails.vi"("Client Name Contains"="EnFlo_Tunnel", "Message"=w462, "Subject"="Zero Heater Power Warning" ("t")) -> ()  [unwired: 2 in, 3 out]
            }
          }
        }
      }
      frame #6 {
        n186 = case shown="True" w495 {
          frame False {
          }
          frame True {
            n187 = Build Array("EnFlo_Tunnel:Heater:Enable") -> (w498:string[])
            n188 = Build Array(0.0) -> (w496:dbl[])
            n189 = call "ASYNC_Adam_server.vi"("Values"=w496, "Channel Names"=w498) -> ()  [unwired: 1 in, 3 out]
          }
        }
      }
    }
  }
